vi "7.vi"() -> ()   [LabVIEW 2021]
uses:
  <vilib>/gmath/NI_AAL_MathFunc.lvlib
panel:
  out "Numeric":i32
  in  "n (to determine n-th prime)":i32
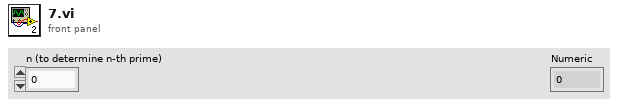
[diagram p1: front panel]
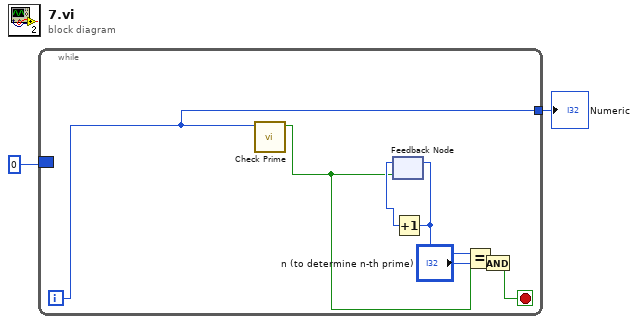
[diagram p0: block diagram]
diagram:
  n1 = while {
    border: 0 -> [_]
    tunnel: [w5] -> w1
    i -> [w5]
    stop <- w4 stop-if-true
    n2 = call <vilib>:"Check Prime.vi"("n"=w5) -> ("prime?"=w3:bool)  [unwired: 10 in]
    n3 = feedback #1() -> (w9:i32)
    n4 = Increment(x=w9) -> (x+1=w8:i32)
    n5 = feedback-in #1(w8, w3) -> ()
    n6 = Equal?(x=w8, y="n (to determine n-th prime)") -> (x = y?=w6:bool)
    n7 = And(x=w6, y=w3) -> (x .and. y?=w4:bool)
  }
  "Numeric" <- w1
